vi "Set Acceleration.vi"(8 "error in (no error)":errorcluster, 10 "acceleration (10000)":u16=10000, 11 "DC Brick in":refnum<class "DC Brick.lvclass">) -> (0 "error out":errorcluster, 3 "DC Brick out":refnum<class "DC Brick.lvclass">)   [LabVIEW 2011, in "Tinkerforge.lvlib" / "DC Brick.lvclass"]
doc: "This VI sets the acceleration of the motor. It is given in velocity/s. An acceleration of 10000 means, that every second the velocity is increased by 10000 (or about 30% duty cycle).\n\nFor example: If the current velocity is 0 and you want to accelerate to a velocity of 16000 (about 50% duty cycle) in 10 seconds, you should set an acceleration of 1600.\n\nIf acceleration is set to 0, there is no speed ramping, i.e. a new velocity is immediately given to the motor.\n\nThe default acceleration is 10000."
uses:
  DC Brick.lvclass
  Device/Device.lvclass
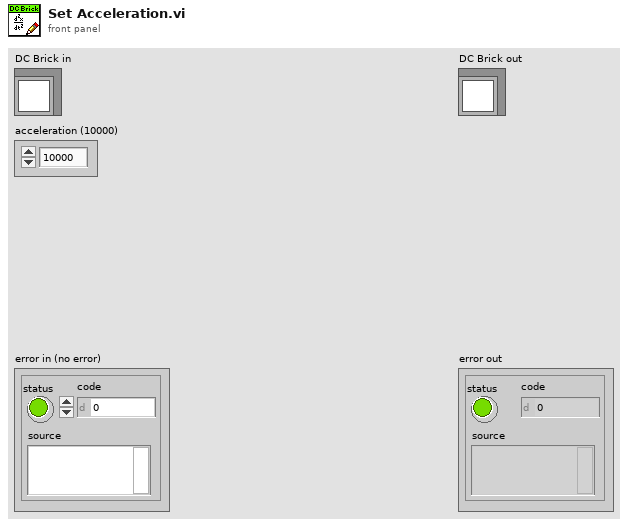
[diagram p1: front panel]
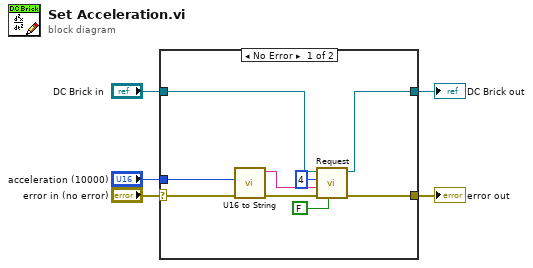
[diagram p0: block diagram]
diagram:
  n1 = case shown="No Error" "error in (no error)" {
    selector: "error in (no error)" -> [w9 w16]
    tunnel: [w10 w16] -> w4
    tunnel: [w13 w15] -> w2
    tunnel: "DC Brick in" -> [w14 w15]
    tunnel: "acceleration (10000)" -> [w8 _]
    frame No Error {
      n2 = call "U16 to String.vi"("Error In"=w9, "U16"=w8) -> ("Error Out"=w7:errorcluster, "String out"=w6:string)  [unwired: 8 in]
      n3 = call "Request.vi"("Response"=FALSE, "error in (no error)"=w7, "Data"=w6, "Function ID"=u8 4, "Device in"=w14) -> ("error out"=w10:errorcluster, "Device out"=w13:refnum<class "DC Brick.lvclass">)  [unwired: 2 in, 3 out]
    }
    frame Error {
    }
  }
  "error out" <- w4
  "DC Brick out" <- w2
